vi "UIRef.vi"(8 "error in":errorcluster, 11 "cRIO in":refnum<class "cRIO.lvclass">) -> (0 "error out":errorcluster, 2 "VI refnum":refnum<vi>, 3 "cRIO out":refnum<class "cRIO.lvclass">)   [LabVIEW 2015, in "cRIO.lvclass"]
uses:
  cRIO.lvclass
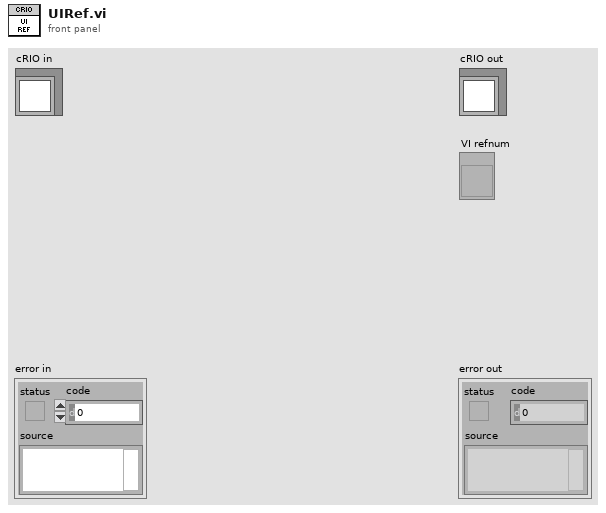
[diagram p1: front panel]
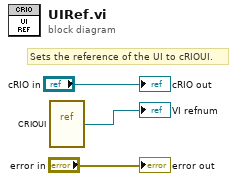
[diagram p0: block diagram]
diagram:
  # "Sets the reference of the UI to cRIOUI."
  n1 = vi-ref "CRIOUI.vi"() -> (→"VI refnum":refnum<vi>)
  "error out" <- "error in"
  "cRIO out" <- "cRIO in"
